vi "add mergin to 2D array.vi"(2 "mergin array":i32[](array[numeric]), 3 "Array in":u8[][](array[numeric])) -> (1 "Array out":u8[][](array[numeric]))   [LabVIEW 2018]
panel:
  # "left (top in image format)"
  # "right (bottom in image format)"
  # "bottom (left in image format)"
  # "top (right in image format)"
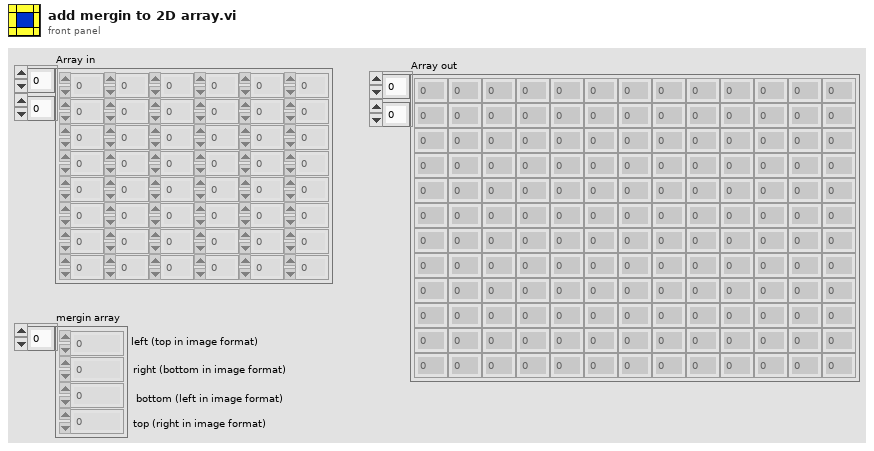
[diagram p1: front panel]
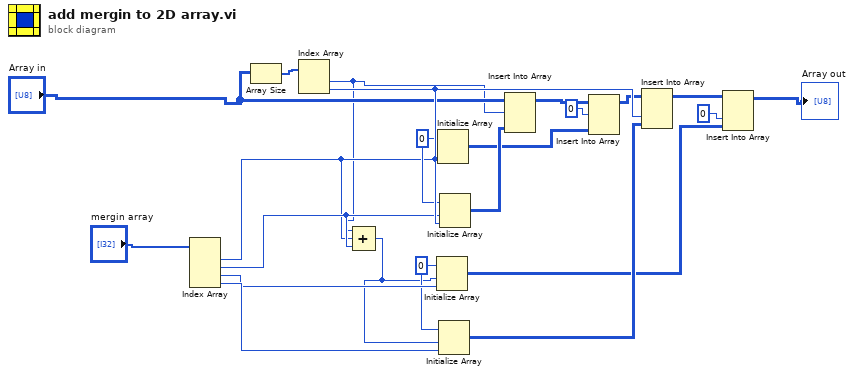
[diagram p0: block diagram]
diagram:
  w16 = u8 0 ("element")
  w13 = u8 0 ("element")
  n1 = Index Array(array="mergin array") -> (element #1=w3:i32, element #2=w4:i32, element #3=w21:i32, element #4=w22:i32)  [unwired: 4 in]
  n2 = Array Size(array="Array in") -> (size(s)=w10:i32[])
  n3 = Index Array(array=w10) -> (element #1=w2:i32, element #2=w18:i32)  [unwired: 2 in]
  n4 = Compound Arithmetic op=ADD(w2, w3, w4) -> (w1:i32)
  n5 = Initialize Array(w16, w1, w21) -> (w17:u8[][])
  n6 = Initialize Array(w13, w3, w18) -> (w12:u8[][])
  n7 = Initialize Array(w16, w1, w22) -> (w19:u8[][])
  n8 = Initialize Array(w13, w4, w18) -> (w14:u8[][])
  n9 = Insert Into Array(array="Array in", index (row)=w2, new element=w14) -> (w8:u8[][])  [unwired: 1 in]
  n10 = Insert Into Array(array=w8, index (row)=0, new element=w12) -> (w7:u8[][])  [unwired: 1 in]
  n11 = Insert Into Array(array=w7, index (col)=w18, new element=w19) -> (w6:u8[][])  [unwired: 1 in]
  n12 = Insert Into Array(array=w6, index (col)=0 ("index (row)"), new element=w17) -> (→"Array out":u8[][])  [unwired: 1 in]
